vi "close_console.vi"(8 "error in (no error)":errorcluster, 11 "console.provider in":refnum<class "console.provider.lvclass">) -> (0 "error out":errorcluster, 3 "console.provider out":refnum<class "console.provider.lvclass">)   [LabVIEW 2021, in "console.provider.lvclass"]
uses:
  console.provider.lvclass
  console_commands.ctl
  console_payload.ctl
  system.logging/log_entry.ctl
  system.logging/severity.ctl
  console.provider.lvclass/console.provider.ctl
  system.logging/system.logging.lvclass
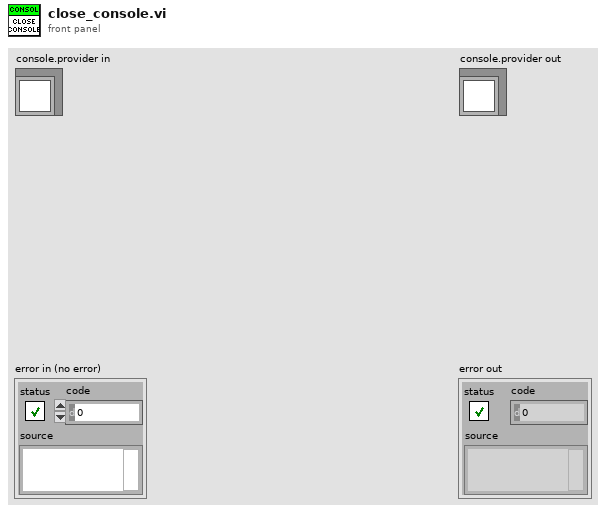
[diagram p1: front panel]
types:
  T1 = typedef "console.provider.lvclass/console_commands.ctl" = enum16{"close", "print"}
  T2 = typedef "console.provider.lvclass/console_payload.ctl" = cluster{"console_cmd":T1, "log":T3}
  T3 = typedef "system.logging.lvclass/log_entry.ctl" = cluster{"severity":T4, "message":string, "origin":string, "datetime":timestamp}
  T4 = typedef "system.logging.lvclass/severity.ctl" = enum8{"trace", "debug", "info", "warning", "error"}
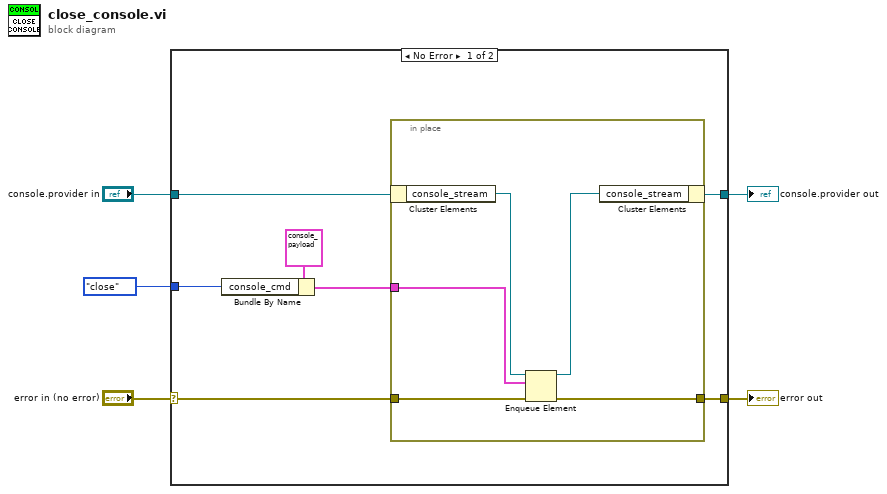
[diagram p0: block diagram]
diagram:
  n1 = case shown="No Error" "error in (no error)" {
    selector: "error in (no error)" -> [w11 w19]
    tunnel: [w9 w19] -> w4
    tunnel: [w10 w18] -> w2
    tunnel: "console.provider in" -> [w12 w18]
    tunnel: console_commands."close" ("console_cmd") -> [w7 _]
    frame No Error {
      n2 = Bundle By Name(cluster=T2 {"console_cmd"=enum."close", "log"={"severity"=enum."trace", "message"="", "origin"="", "datetime"=timestamp(0 s since 1904-01-01)}} ("console_payload"), "console_cmd"=w7) -> (w6:T2)
      n3 = in-place {
        in-place-border: w11 -> [w17]
        in-place-border: [w14] -> w9
        in-place-border: w6 -> [w13]
        n4 = in-place-cluster #1(w12) -> ("console_stream"=w16:refnum<queue>)
        n5 = Enqueue Element(queue=w16, element=w13, error in (no error)=w17) -> (queue out=w15:refnum<queue>, error out=w14:errorcluster)  [unwired: 1 in, 1 out]
        n6 = in-place-cluster #1("console_stream"=w15) -> (w10:refnum<class "console.provider.lvclass">)
      }
    }
    frame Error {
    }
  }
  "error out" <- w4
  "console.provider out" <- w2
